vi "Pre Launch Init.vi"(11 "UI Main in":refnum<class "UI Main.lvclass">) -> (0 "error out":errorcluster, 3 "UI Main out":refnum<class "UI Main.lvclass">)   [LabVIEW 2020, in "UI Main.lvlib" / "UI Main.lvclass"]
doc: "(<B>Filename</B>: Actor Framework.lvlib:Actor.lvclass:Pre Launch Init.vi)\n\nDefines behavior that occurs after the Launch Nested Actor method is invoked but before the actor's Actor Core method begins running.\n\nBy default, this method does nothing. A descendant class may override it to define behavior."
uses:
  UI Main.lvclass
  Sub Panel.ctl
  UI Main.lvclass/UI Main.ctl
  <vilib>/ActorFramework/Actor/Actor.lvclass
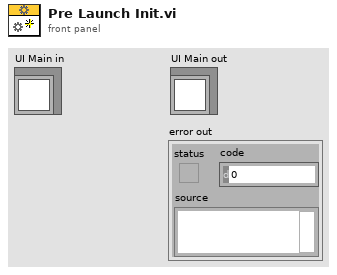
[diagram p1: front panel]
types:
  T1 = typedef "UI Main.lvlib/UI Main.lvclass/Sub Panel.ctl" = cluster{"Clone Name":string, "UI Section":string}
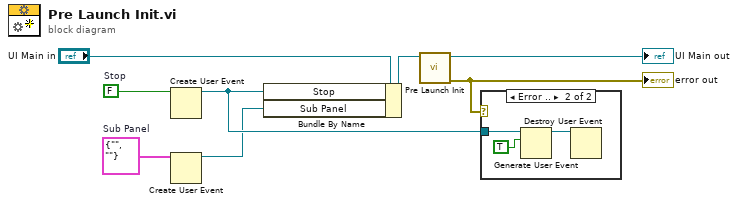
[diagram p0: block diagram]
diagram:
  w2 = T1 {"Clone Name"="", "UI Section"=""}  # Sub Panel
  w7 = FALSE  # Stop
  n1 = Create User Event(user event datatype=w7) -> (user event=w3:refnum<user-event>)  [unwired: 1 in, 1 out]
  n2 = Create User Event(user event datatype=w2) -> (user event=w1:refnum<user-event>)  [unwired: 1 in, 1 out]
  n3 = Bundle By Name(cluster="UI Main in", "Stop"=w3, "Sub Panel"=w1) -> (w5:refnum<class "UI Main.lvclass">)
  n4 = call-parent "Pre Launch Init.vi"("Actor in"=w5) -> ("error out"=w4:errorcluster, "Actor out"=→"UI Main out":refnum<class "UI Main.lvclass">)  [unwired: 9 in]
  "error out" <- w4
  n5 = case shown="Error .." w4 {
    tunnel: w3 -> [_ w11]
    frame No Error {
    }
    frame Error {
      n6 = Generate User Event(user event=w11, event data cluster=TRUE ("event data")) -> (user event out=w9:refnum<user-event>)  [unwired: 2 in, 1 out]
      n7 = Destroy User Event(user event=w9) -> ()  [unwired: 1 in, 1 out]
    }
  }
